vi "String To GUID Cluster.vi"(4 "error in (no error)":errorcluster, 7 "Input String":string) -> (0 "error out":errorcluster, 3 "GUID":T1 {"GUID1" format="%.0x"; "GUID2" format="%.0x"; "GUID3" format="%.0x"; "GUID4"."GUID4[0]" format="%.0x"; "GUID4"."GUID4[1]" format="%.0x"; "GUID4"."GUID4[2]" format="%.0x"; "GUID4"."GUID4[3]" format="%.0x"; "GUID4"."GUID4[4]" format="%.0x"; "GUID4"."GUID4[5]" format="%.0x"; "GUID4"."GUID4[6]" format="%.0x"; "GUID4"."GUID4[7]" format="%.0x"})   [LabVIEW 2012]
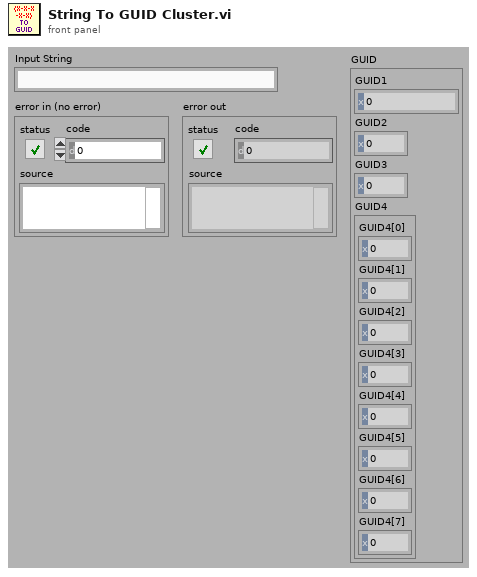
[diagram p1: front panel]
types:
  T1 = cluster{"GUID1":u32, "GUID2":u16, "GUID3":u16, "GUID4":cluster{"GUID4[0]":u8, "GUID4[1]":u8, "GUID4[2]":u8, "GUID4[3]":u8, "GUID4[4]":u8, "GUID4[5]":u8, "GUID4[6]":u8, "GUID4[7]":u8}}
  T2 = cluster{"GUID4[0]":u8, "GUID4[1]":u8, "GUID4[2]":u8, "GUID4[3]":u8, "GUID4[4]":u8, "GUID4[5]":u8, "GUID4[6]":u8, "GUID4[7]":u8}
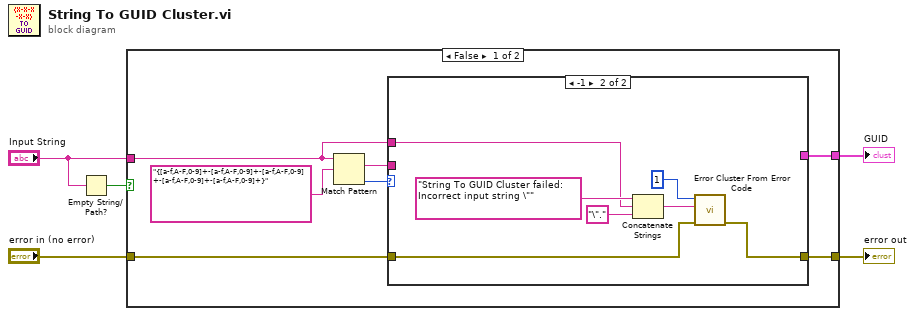
[diagram p0: block diagram]
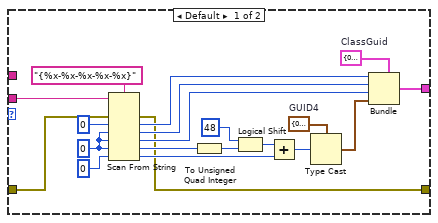
[diagram p2: hidden frame]
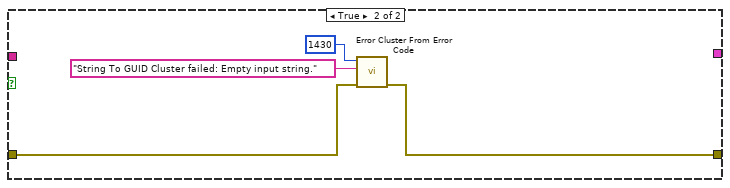
[diagram p3: hidden frame]
diagram:
  n1 = Empty String/Path?(string/path="Input String") -> (empty?=w5:bool)
  n2 = case shown="False" w5 {
    tunnel: "Input String" -> [w6 _]
    tunnel: "error in (no error)" -> [w9 w41]
    tunnel: [w8 _] -> w2
    tunnel: [w7 w40] -> w1
    frame False {
      n3 = Match Pattern(string=w6, regular expression="{[a-f,A-F,0-9]+-[a-f,A-F,0-9]+-[a-f,A-F,0-9]+-[a-f,A-F,0-9]+-[a-f,A-F,0-9]+}") -> (match substring=w10:string, offset past match=w11:i32)  [unwired: 1 in, 2 out]
      n4 = case shown="-1" w11 {
        tunnel: w10 -> [w31 _]
        tunnel: w9 -> [w15 w36]
        tunnel: [w14 _] -> w8
        tunnel: [w13 w34] -> w7
        tunnel: w6 -> [_ w33]
        frame Default {
          w16 = T1 {"GUID1"=0, "GUID2"=0, "GUID3"=0, "GUID4"={"GUID4[0]"=0, "GUID4[1]"=0, "GUID4[2]"=0, "GUID4[3]"=0, "GUID4[4]"=0, "GUID4[5]"=0, "GUID4[6]"=0, "GUID4[7]"=0}}  # ClassGuid
          w21 = T2 {"GUID4[0]"=0, "GUID4[1]"=0, "GUID4[2]"=0, "GUID4[3]"=0, "GUID4[4]"=0, "GUID4[5]"=0, "GUID4[6]"=0, "GUID4[7]"=0}  # GUID4
          w29 = u16 0 ("default value 2")
          n5 = Scan From String(format string="{%x-%x-%x-%x-%x}", input string=w31, error in=w15, default 1=u32 0 ("default value 1"), default 2=w29, default 3=w29, default 4=w29, default 5=u64 0 ("default value 5")) -> (error out=w13:errorcluster, output 1=w20:u32, output 2=w19:u16, output 3=w18:u16, output 4=w25:u16, output 5=w27:u64)  [unwired: 1 in, 2 out]
          n6 = To Unsigned Quad Integer(1:w25) -> (0:w24:u64)
          n7 = Logical Shift(y=i16 48, x=w24) -> (x << y=w22:u64)
          n8 = Add(x=w22, y=w27) -> (x+y=w26:u64)
          n9 = Type Cast(type=w21, x=w26) -> (*(type *) &x=w17:T2)
          n10 = Bundle(cluster=w16, "GUID1"=w20, "GUID2"=w19, "GUID3"=w18, "GUID4"=w17) -> (w14:T1)
        }
        frame -1 {
          n11 = Concatenate Strings("String To GUID Cluster failed: Incorrect input string \"" ("error message (\"\")"), w33, "\"." ("string")) -> (w35:string)
          n12 = call <vilib>:"Error Cluster From Error Code.vi"("error in (no error)"=w36, "error message (\"\")"=w35, "error code (0)"=1) -> ("error out"=w34:errorcluster)  [unwired: 6 in]
        }
      }
    }
    frame True {
      n13 = call <vilib>:"Error Cluster From Error Code.vi"("error in (no error)"=w41, "error message (\"\")"="String To GUID Cluster failed: Empty input string." ("error message (\"\")"), "error code (0)"=1430) -> ("error out"=w40:errorcluster)  [unwired: 6 in]
    }
  }
  "error out" <- w1
  "GUID" <- w2
